vi "Get Bounds (Integer).vi"(8 "error in (no error)":errorcluster, 10 "Feature":string, 11 "Camera in":refnum<class "Camera.lvclass">) -> (0 "error out":errorcluster, 1 "Max":i64, 2 "Min":i64, 3 "Camera":refnum<class "Camera.lvclass">)   [LabVIEW 2020, in "Camera.lvclass"]
uses:
  Camera.lvclass
  Camera.lvclass/Camera.ctl
  bin/gindustrialcam_32-1.dll
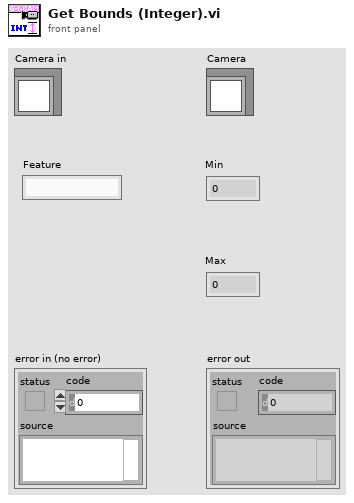
[diagram p1: front panel]
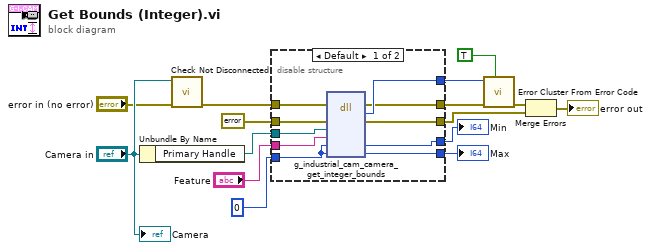
[diagram p0: block diagram]
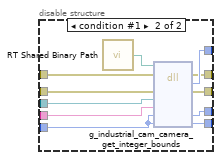
[diagram p2: hidden frame]
diagram:
  n1 = Unbundle By Name("Camera in") -> ("Primary Handle"=w10:refnum<data-value>)
  n2 = call "Check Not Disconnected.vi"("error in (no error)"="error in (no error)", "Camera in"="Camera in") -> ("error out"=w11:errorcluster)  [unwired: 9 in]
  n3 = disable-structure shown="Default" {
    disable-tunnel: [w25 w36] -> w12
    disable-tunnel: w11 -> [w24 w35]
    disable-tunnel: w10 -> [w23 w34]
    disable-tunnel: errorcluster {"status"=FALSE, "code"=0, "source"=""} ("error constant") -> [w22 w33]
    disable-tunnel: [w21 w32] -> w7
    disable-tunnel: [w20 w31] -> w5
    disable-tunnel: [w19 w30] -> w4
    disable-tunnel: [w18 w29] -> w3
    disable-tunnel: i64 0 ("Value In") -> [w17 w28]
    disable-tunnel: "Feature" -> [w16 w27]
    frame condition #0 (active) {
      n4 = dll-call lib="C:/serenial/lib/g-industrial-camera/LabVIEW/g_industrial_cam/bin/gindustrialcam_*-1.*" fn="g_industrial_cam_camera_get_integer_bounds"(error in=w24, "err"=w22, "edvr"=w23, "feature"=w16, "min"=w17, "max"=w17) -> (error out=w19:errorcluster, "Mg_Error"=w20:i32, "err"=w21:errorcluster, "min"=w25:i64, "max"=w18:i64)  [unwired: 4 in, 1 out]
    }
    frame condition #1 {
      n5 = call "RT Shared Binary Path.vi"() -> ("Path"=w26:path)
      n6 = dll-call lib="C:/serenial/lib/g-industrial-camera/LabVIEW/g_industrial_cam/bin/gindustrialcam_*-1.*" fn="g_industrial_cam_camera_get_integer_bounds"(path in=w26, error in=w35, "err"=w33, "edvr"=w34, "feature"=w27, "min"=w28, "max"=w28) -> (error out=w30:errorcluster, "Mg_Error"=w31:i32, "err"=w32:errorcluster, "min"=w36:i64, "max"=w29:i64)  [unwired: 3 in, 1 out]
    }
  }
  "Min" <- w12
  "Max" <- w3
  n7 = call <vilib>:"Error Cluster From Error Code.vi"("show call chain? (False)"=TRUE, "error in (no error)"=w4, "error code (0)"=w5) -> ("error out"=w6:errorcluster)  [unwired: 6 in]
  n8 = Merge Errors(w6, w7) -> (→"error out":errorcluster)
  "Camera" <- "Camera in"
